vi "manipulating json documents.vi"() -> ()   [LabVIEW 2016]
uses:
  API/JSON Document Class/json insert/json Insert - String Path.vi
  API/JSON Document Class/json to string/json To Minimized String - string path.vi
  API/JSON Document Class/json clone/json Clone - string path.vi
  API/JSON Document Class/JSON Document.lvclass
panel:
  out "new JSON":string
  out "branch a after b mod":string
  out "b modded after sub":string
  out "A with B as sub":string
  out "branch B":string
  out "branch A":string
  # "create new JSON"
  # "insert B into A. B is deep-copied\nback on to A"
  # "clone JSON, and modify\neach branch"
  # "we can modify B and A remains\nunchanged."
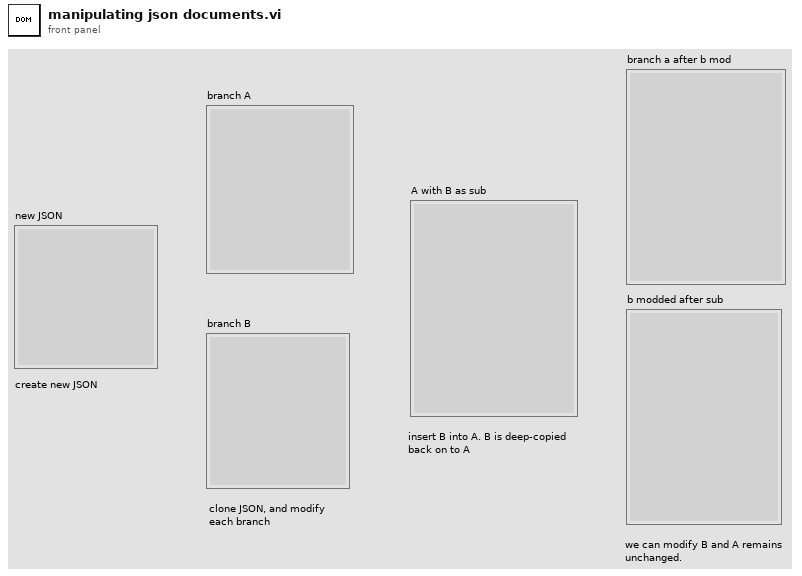
[diagram p1: front panel]
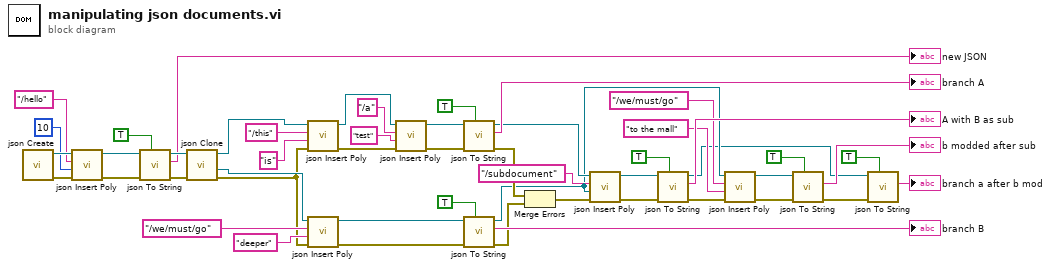
[diagram p0: block diagram]
diagram:
  n1 = call "json Create.vi"() -> ("error out"=w24:errorcluster, "JSON Document out"=w50:refnum<class "JSON Document.lvclass">)  [unwired: 10 in]
  n2 = call-poly "json Insert Poly.vi"("error in (no error)"=w24, "anything"=10, "path"="/hello", "JSON Document in"=w50) -> ("error out"=w3:errorcluster, "JSON Document out"=w5:refnum<class "JSON Document.lvclass">)  [unwired: 5 in, 1 out]
  n3 = call-poly "json To String.vi"("pretty print?"=TRUE, "error in (no error)"=w3, "JSON Document in"=w5) -> ("error out"=w2:errorcluster, "json string"=→"new JSON":string, "JSON Document out"=w4:refnum<class "JSON Document.lvclass">)  [unwired: 6 in]
  n4 = call-poly "json Clone.vi"("error in (no error)"=w2, "JSON Document in"=w4) -> ("error out"=w23:errorcluster, 1:"JSON Document out"=w39:refnum<class "JSON Document.lvclass">, 3:"JSON Document out"=w47:refnum<class "JSON Document.lvclass">)  [unwired: 7 in]
  n5 = call-poly "json Insert Poly.vi"("error in (no error)"=w23, "anything"="is" ("path"), "path"="/this", "JSON Document in"=w47) -> ("error out"=w22:errorcluster, "JSON Document out"=w46:refnum<class "JSON Document.lvclass">)  [unwired: 5 in, 1 out]
  n6 = call-poly "json Insert Poly.vi"("error in (no error)"=w23, "anything"="deeper" ("path"), "path"="/we/must/go", "JSON Document in"=w39) -> ("error out"=w34:errorcluster, "JSON Document out"=w33:refnum<class "JSON Document.lvclass">)  [unwired: 5 in, 1 out]
  n7 = call-poly "json Insert Poly.vi"("error in (no error)"=w22, "anything"="test" ("path"), "path"="/a", "JSON Document in"=w46) -> ("error out"=w37:errorcluster, "JSON Document out"=w36:refnum<class "JSON Document.lvclass">)  [unwired: 5 in, 1 out]
  n8 = call-poly "json To String.vi"("pretty print?"=TRUE, "error in (no error)"=w37, "JSON Document in"=w36) -> ("error out"=w21:errorcluster, "json string"=→"branch A":string, "JSON Document out"=w30:refnum<class "JSON Document.lvclass">)  [unwired: 6 in]
  n9 = call-poly "json To String.vi"("pretty print?"=TRUE, "error in (no error)"=w34, "JSON Document in"=w33) -> ("error out"=w20:errorcluster, "json string"=→"branch B":string, "JSON Document out"=w13:refnum<class "JSON Document.lvclass">)  [unwired: 6 in]
  n10 = Merge Errors(w21, w20) -> (w19:errorcluster)
  n11 = call-poly "json Insert Poly.vi"("error in (no error)"=w19, "anything"=w13, "path"="/subdocument", "JSON Document in"=w30) -> ("error out"=w27:errorcluster, "JSON Document out"=w25:refnum<class "JSON Document.lvclass">)  [unwired: 5 in, 1 out]
  n12 = call-poly "json To String.vi"("pretty print?"=TRUE, "error in (no error)"=w27, "JSON Document in"=w25) -> ("error out"=w12:errorcluster, "json string"=→"A with B as sub":string, "JSON Document out"=w8:refnum<class "JSON Document.lvclass">)  [unwired: 6 in]
  n13 = call-poly "json Insert Poly.vi"("error in (no error)"=w12, "anything"="to the mall" ("path"), "path"="/we/must/go", "JSON Document in"=w13) -> ("error out"=w14:errorcluster, "JSON Document out"=w15:refnum<class "JSON Document.lvclass">)  [unwired: 5 in, 1 out]
  n14 = call-poly "json To String.vi"("pretty print?"=TRUE, "error in (no error)"=w14, "JSON Document in"=w15) -> ("error out"=w9:errorcluster, "json string"=→"b modded after sub":string)  [unwired: 6 in, 1 out]
  n15 = call-poly "json To String.vi"("pretty print?"=TRUE, "error in (no error)"=w9, "JSON Document in"=w8) -> ("json string"=→"branch a after b mod":string)  [unwired: 6 in, 2 out]
